vi "OverwriteChannel.vi"(8 "error in (no error)":errorcluster, 9 "ChannelIndex":i32, 10 "Channel":T1, 11 "DCM-DSI-HW in":refnum<class "DCM-DSI.lvclass">) -> (0 "error out":errorcluster, 3 "DCM-DSI-HW out":refnum<class "DCM-DSI.lvclass">)   [LabVIEW 2016, in "DCM-DSI.lvclass"]
uses:
  DCM-DSI.lvclass
  Shared/Typedefs/Engine-Channel.ctl
  DCM-DSI.lvclass/DCM-DSI.ctl
  Shared/DSI-Shared.lvlib
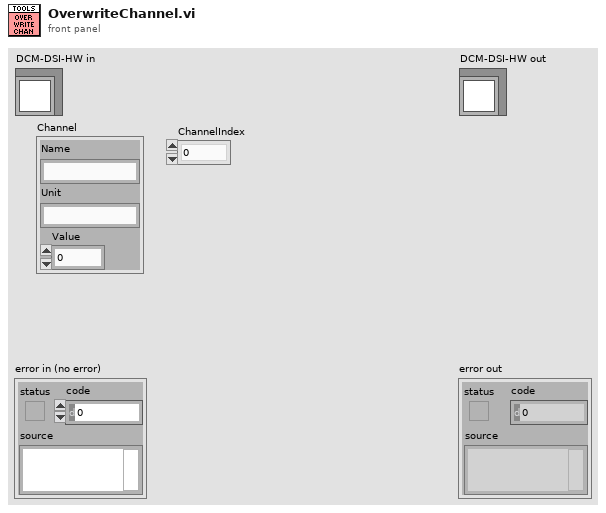
[diagram p1: front panel]
types:
  T1 = typedef "DSI-Shared.lvlib/Engine-Channel.ctl" = cluster{"Name":string, "Unit":string, "Value":sgl}
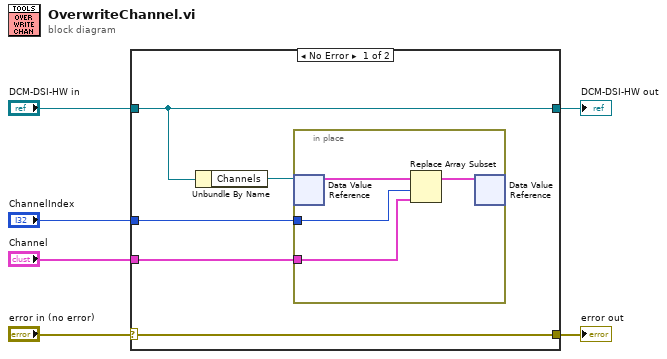
[diagram p0: block diagram]
diagram:
  n1 = case shown="No Error" "error in (no error)" {
    selector: "error in (no error)" -> [w11 w17]
    tunnel: [w11 w17] -> w5
    tunnel: [w9 w16] -> w3
    tunnel: "DCM-DSI-HW in" -> [w9 w16]
    tunnel: "Channel" -> [w8 _]
    tunnel: "ChannelIndex" -> [w7 _]
    frame No Error {
      n2 = Unbundle By Name(w9) -> ("Channels"=w10:refnum<data-value>)
      n3 = in-place {
        in-place-border: w8 -> [w13]
        in-place-border: w7 -> [w12]
        n4 = in-place-dvr #1(w10) -> (w15:T1[])  [unwired: 1 out]
        n5 = Replace Array Subset(array=w15, new element=w13, index=w12) -> (w14:T1[])
        n6 = in-place-dvr #1(w14) -> ()  [unwired: 2 out]
      }
    }
    frame Error {
    }
  }
  "error out" <- w5
  "DCM-DSI-HW out" <- w3
